vi "AVI Video-Close files.vi"(8 "error in (no error)":errorcluster) -> (0 "error out (pass through)":errorcluster)   [LabVIEW 2017]
uses:
  Typedefs/Channel Selector.ctl
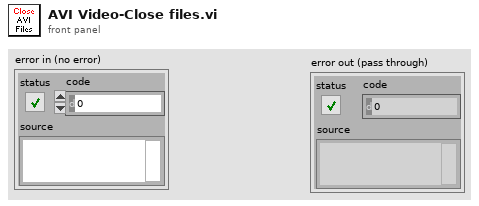
[diagram p1: front panel]
types:
  T1 = typedef "Channel Selector.ctl" = enum16{"Red Channel", "Green Channel", "Blended"}
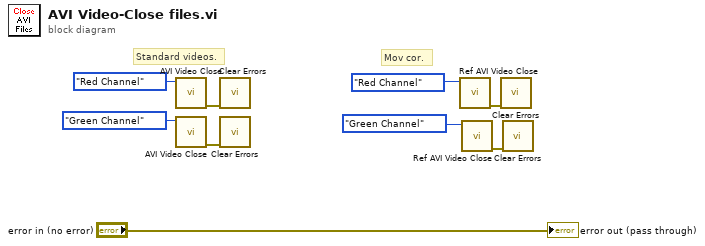
[diagram p0: block diagram]
diagram:
  # "Standard videos."
  # "Mov cor."
  n1 = call "AVI Video Close.vi"("Channel"=Channel_Selector."Red Channel") -> ("error out"=w8:errorcluster)  [unwired: 10 in]
  n2 = call "AVI Video Close.vi"("Channel"=Channel_Selector."Green Channel") -> ("error out"=w9:errorcluster)  [unwired: 10 in]
  n3 = call <vilib>:"Clear Errors.vi"("error in (no error)"=w8) -> ()  [unwired: 5 in, 2 out]
  n4 = call <vilib>:"Clear Errors.vi"("error in (no error)"=w9) -> ()  [unwired: 5 in, 2 out]
  n5 = call "Ref AVI Video Close.vi"("Channel"=Channel_Selector."Red Channel") -> ("error out"=w2:errorcluster)  [unwired: 10 in]
  n6 = call "Ref AVI Video Close.vi"("Channel"=Channel_Selector."Green Channel") -> ("error out"=w4:errorcluster)  [unwired: 10 in]
  n7 = call <vilib>:"Clear Errors.vi"("error in (no error)"=w2) -> ()  [unwired: 5 in, 2 out]
  n8 = call <vilib>:"Clear Errors.vi"("error in (no error)"=w4) -> ()  [unwired: 5 in, 2 out]
  "error out (pass through)" <- "error in (no error)"
